vi "SEN_Loop.vi"() -> ()   [LabVIEW 2020, in "JoystickController_SEN.lvlib"]
uses:
  JoystickController_SEN.lvlib
  ENUM_SEN_State.ctl
  <vilib>/Rock Robotics/WPI/Joystick/WPI_JoystickDevRef.ctl
  <vilib>/Rock Robotics/WPI/Joystick/WPI_JoystickDeviceEnum.ctl
  ENUM_SEN_Action.ctl
  Utility/Global_STOP.vi
  Global_SEN_Data Out.vi
panel:
  out "Input Bool Data":bool
  out "Output DBL Data":dbl
  out "Cycle Time (S)":dbl format="%.3g"
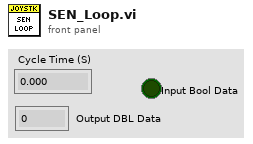
[diagram p1: front panel]
types:
  T1 = typedef "WPI_JoystickDevRef.ctl" = cluster{"Device":T2}
  T2 = typedef "WPI_JoystickDeviceEnum.ctl" = enum16{"USB 0", "USB 1", "USB 2", "USB 3", "USB 4", "USB 5"}
  T3 = typedef "JoystickController_SEN.lvlib/ENUM_SEN_State.ctl" = enum16{"Startup", "Enable", "Shutdown"}
  T4 = typedef "JoystickController_SEN.lvlib/ENUM_SEN_Action.ctl" = enum16{"No Action", "Reset Time", "Read Enable", "Read Disable"}
  T5 = cluster{"Sensor Ref 1":T1, "Sensor Ref 0":T1, "State":T3, "Previous State":T3, "Current Time":timestamp, "Previous Time":timestamp, "Start Time":timestamp, "Target Time (ms)":u32, "Cycle Time(S)":dbl, "SEN Input":bool, "SEN Output DBL":dbl, "Read Enable":bool, "Axes 0":dbl[], "Buttons 0":bool[], "POVs 0":i16[], "Axes 1":dbl[], "Buttons 1":bool[], "POVs 1":i16[]}
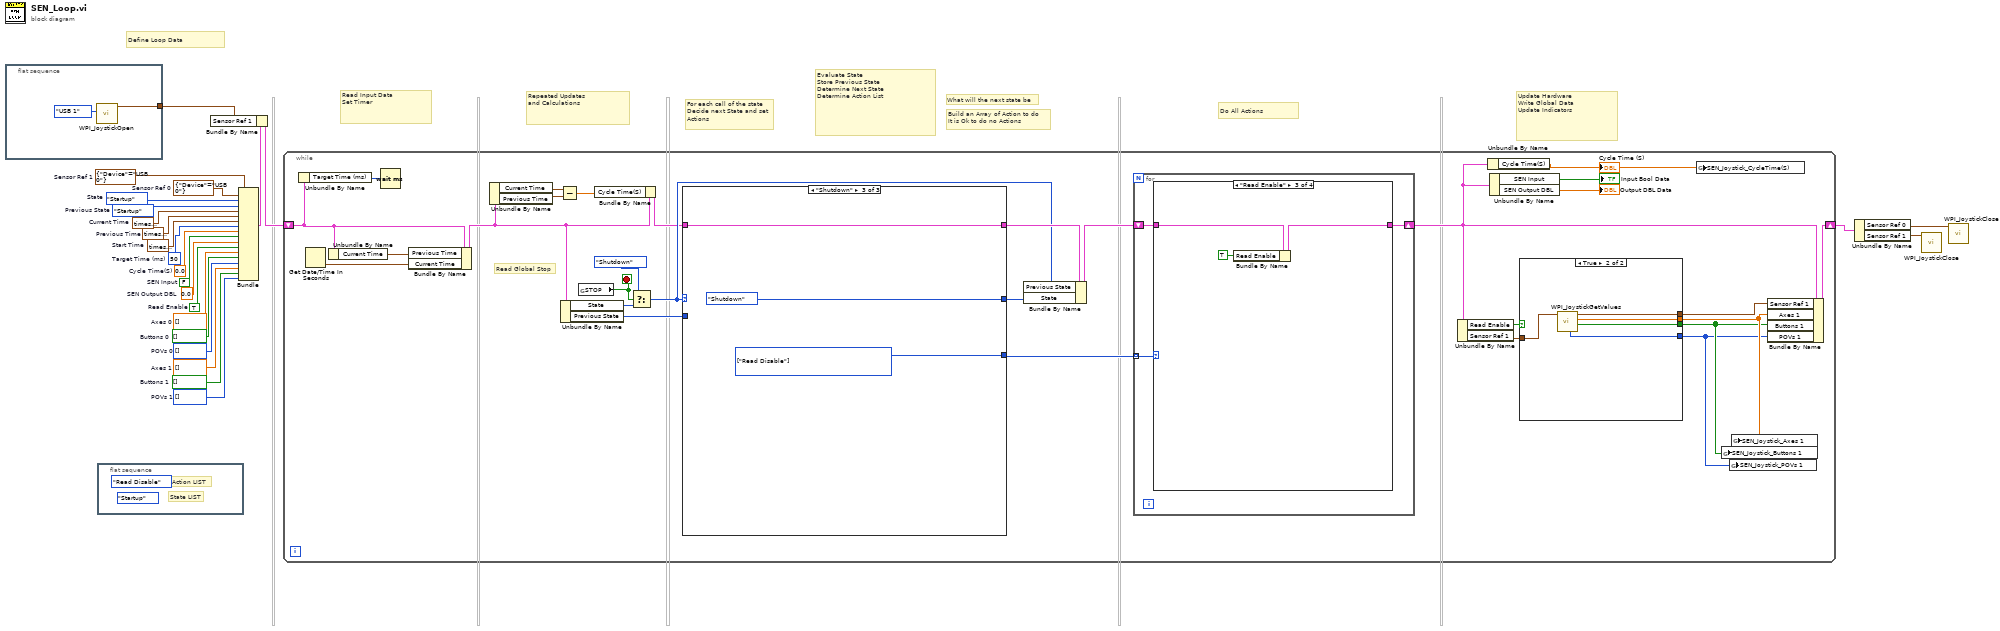
[diagram p0: block diagram]
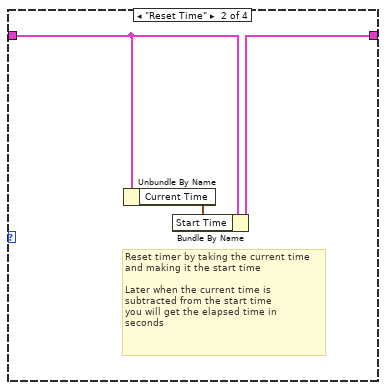
[diagram p4: hidden frame]
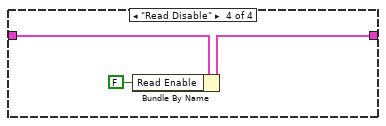
[diagram p5: hidden frame]
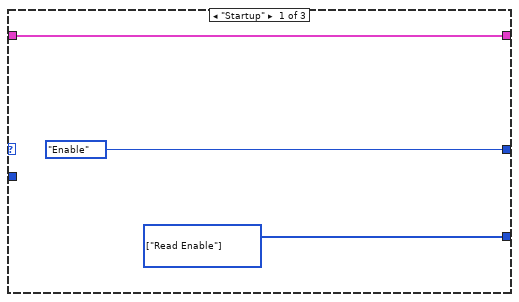
[diagram p6: hidden frame]
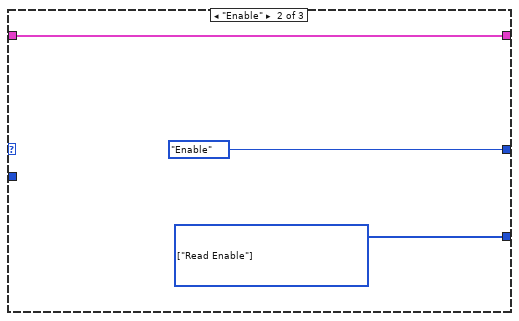
[diagram p7: hidden frame]
diagram:
  w1 = T1 {"Device"=enum."USB 0"}  # Sensor Ref 0
  w2 = T1 {"Device"=enum."USB 0"}  # Sensor Ref 1
  w5 = i16[] []  # POVs 1
  w6 = bool[] []  # Buttons 1
  w7 = dbl[] []  # Axes 1
  w8 = i16[] []  # POVs 0
  w9 = bool[] []  # Buttons 0
  w10 = dbl[] []  # Axes 0
  w14 = TRUE  # Read Enable
  w16 = 0.0  # Cycle Time(S)
  w17 = ENUM_SEN_State."Startup"  # Previous State
  w18 = timestamp(0 s since 1904-01-01)  # Previous Time
  w19 = u32 50  # Target Time (ms)
  w20 = 0.0  # SEN Output DBL
  w21 = FALSE  # SEN Input
  w22 = timestamp(0 s since 1904-01-01)  # Start Time
  w23 = timestamp(0 s since 1904-01-01)  # Current Time
  w24 = ENUM_SEN_State."Startup"  # State
  # "Build an Array of Action to do\nIt is Ok to do no Actions"
  # "What will the next state be"
  # "For each call of the state\nDecide next State and set\nActions"
  # "Define Loop Data"
  # "Repeated Updates\nand Calculations"
  # "Read Input Data\nSet Timer"
  # "Evaluate State\nStore Previous State\nDetermine Next State\nDetermine Action List"
  # "Do All Actions"
  # "Update Hardware\nWrite Global Data\nUpdate Indicators"
  n1 = flat-sequence {
    tunnel: [w25] -> w11
    frame #0 {
      n2 = call <vilib>:"WPI_JoystickOpen.vi"("JoystickDevice"=WPI_JoystickDeviceEnum."USB 1") -> ("JoystickDevRef"=w25:T1)  [unwired: 10 in]
    }
  }
  n3 = flat-sequence {
    frame #0 {
      (unwired) ENUM_SEN_State."Startup" ("State")
      (unwired) ENUM_SEN_Action."Read Disable" ("Action")
      # "State LIST"
      # "Action LIST"
    }
  }
  n4 = Bundle("Sensor Ref 1"=w2, "Sensor Ref 0"=w1, "State"=w24, "Previous State"=w17, "Current Time"=w23, "Previous Time"=w18, "Start Time"=w22, "Target Time (ms)"=w19, "Cycle Time(S)"=w16, "SEN Input"=w21, "SEN Output DBL"=w20, "Read Enable"=w14, "Axes 0"=w10, "Buttons 0"=w9, "POVs 0"=w8, "Axes 1"=w7, "Buttons 1"=w6, "POVs 1"=w5) -> (w13:T5)  [unwired: 1 in]
  n5 = Bundle By Name(cluster=w13, "Sensor Ref 1"=w11) -> (w12:T5)
  n6 = while {
    shift-right: [w33] -> w15
    shift-left: w12 -> [w46]
    stop <- w51 stop-if-true
    # "Read Global Stop"
    n7 = Unbundle By Name(w46) -> ("Target Time (ms)"=w48:u32)
    n8 = Get Date/Time In Seconds() -> (seconds since 1Jan1904=w55:timestamp)
    n9 = Unbundle By Name(w46) -> ("Current Time"=w47:timestamp)
    n10 = Wait (ms)(milliseconds to wait=w48) -> ()  [unwired: 1 out]
    n11 = Bundle By Name(cluster=w46, "Previous Time"=w47, "Current Time"=w55) -> (w40:T5)
    n12 = Unbundle By Name(w40) -> ("Current Time"=w41:timestamp, "Previous Time"=w42:timestamp)
    n13 = Subtract(x=w41, y=w42) -> (x-y=w38:dbl)
    n14 = Unbundle By Name(w40) -> ("State"=w49:T3, "Previous State"=w45:T3)
    n15 = global read "Global_STOP.vi" "STOP"() -> (w51:bool)
    n16 = Bundle By Name(cluster=w40, "Cycle Time(S)"=w38) -> (w39:T5)
    n17 = Select(t=ENUM_SEN_State."Shutdown" ("State"), s=w51, f=w49) -> (s? t:f=w43:T3)
    n18 = case shown="\"Shutdown\"" w43 {
      tunnel: w39 -> [w77 w78 w83]
      tunnel: [w77 w78 w83] -> w53
      tunnel: [ENUM_SEN_State."Enable" ("State") ENUM_SEN_State."Enable" ("State") ENUM_SEN_State."Shutdown" ("State")] -> w52
      tunnel: [w76 w80 w81] -> w37
      tunnel: w45 -> [_ _ _]
      frame "Startup" {
        w76 = T4[] [enum."Read Enable"] items=["No Action", "Reset Time", "Read Enable", "Read Disable"] ("Actions")
      }
      frame "Enable" {
        w80 = T4[] [enum."Read Enable"] items=["No Action", "Reset Time", "Read Enable", "Read Disable"] ("Actions")
      }
      frame "Shutdown" {
        w81 = T4[] [enum."Read Disable"] items=["No Action", "Reset Time", "Read Enable", "Read Disable"] ("Actions")
      }
    }
    n19 = Bundle By Name(cluster=w53, "Previous State"=w43, "State"=w52) -> (w54:T5)
    n20 = for {
      tunnel: w37 -> [w64] mode=indexing
      shift-right: [w63] -> w34
      shift-left: w54 -> [w62]
      n21 = case shown="\"Read Enable\"" w64 {
        tunnel: w62 -> [w65 w68 w71 w74]
        tunnel: [w65 w67 w70 w73] -> w63
        frame "No Action" {
        }
        frame "Reset Time" {
          # "Reset timer by taking the current time\nand making it the start time\n\nLater when the current time is \nsubtracted from the start time\nyou will get the elapsed time in \nseconds"
          n22 = Unbundle By Name(w68) -> ("Current Time"=w66:timestamp)
          n23 = Bundle By Name(cluster=w68, "Start Time"=w66) -> (w67:T5)
        }
        frame "Read Enable" {
          n24 = Bundle By Name(cluster=w71, "Read Enable"=TRUE) -> (w70:T5)
        }
        frame "Read Disable" {
          n25 = Bundle By Name(cluster=w74, "Read Enable"=FALSE) -> (w73:T5)
        }
      }
    }
    n26 = Unbundle By Name(w34) -> ("Read Enable"=w31:bool, "Sensor Ref 1"=w35:T1)
    n27 = Unbundle By Name(w34) -> ("Cycle Time(S)"=w32:dbl)
    "Cycle Time (S)" <- w32
    n28 = Unbundle By Name(w34) -> ("SEN Input"=→"Input Bool Data":bool, "SEN Output DBL"=→"Output DBL Data":dbl)
    n29 = case shown="True" w31 {
      tunnel: w35 -> [w56 w61]
      tunnel: [w56 w60] -> w30
      tunnel: [_ w59] -> w29
      tunnel: [_ w58] -> w28
      tunnel: [_ w57] -> w27
      frame False {
      }
      frame True {
        n30 = call <vilib>:"WPI_JoystickGetValues.vi"("JoystickDevRef"=w61) -> ("Buttons"=w58:bool[], "Axes"=w59:dbl[], "JoystickDevRef"=w60:T1, "POVs"=w57:i16[])  [unwired: 6 in, 1 out]
      }
    }
    n31 = global write "Global_SEN_Data Out.vi" "SEN_Joystick_CycleTime(S)"(w32) -> ()
    n32 = global write "Global_SEN_Data Out.vi" "SEN_Joystick_Buttons 1"(w28) -> ()
    n33 = global write "Global_SEN_Data Out.vi" "SEN_Joystick_POVs 1"(w27) -> ()
    n34 = global write "Global_SEN_Data Out.vi" "SEN_Joystick_Axes 1"(w29) -> ()
    n35 = Bundle By Name(cluster=w34, "Sensor Ref 1"=w30, "Axes 1"=w29, "Buttons 1"=w28, "POVs 1"=w27) -> (w33:T5)
  }
  n36 = Unbundle By Name(w15) -> ("Sensor Ref 0"=w4:T1, "Sensor Ref 1"=w3:T1)
  n37 = call <vilib>:"WPI_JoystickClose.vi"("JoystickDevRef"=w3) -> ()  [unwired: 11 in]
  n38 = call <vilib>:"WPI_JoystickClose.vi"("JoystickDevRef"=w4) -> ()  [unwired: 11 in]
